vi "FIFO_96ch_Clear.vi"(3 "error in":errorcluster, 5 "FPGA VI Reference In":T1) -> (0 "error out":errorcluster, 2 "FPGA VI Reference Out":T1)   [LabVIEW 2011]
uses:
  FPGA_reference.ctl
  <vilib>/Utility/error.llb/Error Cluster From Error Code.vi
  <vilib>/rvi/errors/niLvFpgaAdjustHostInterfaceError.vi
  <vilib>/rvi/interface/nirviMethod/nirviMethod.xnode
  FPGA Bitfiles/FPGA96chmodular3_FPGATarget_fpga8ch-Main_90409DC7.lvbitx
  fpga_8ch-Main.vi
  <vilib>/FPGAPlugInAG/PXI-7813R/niLvFpga_ReadFifo_PXI-7813R.vi
  <vilib>/rvi/errors/niLvFpgaMergeErrorWithErrorCode.vi
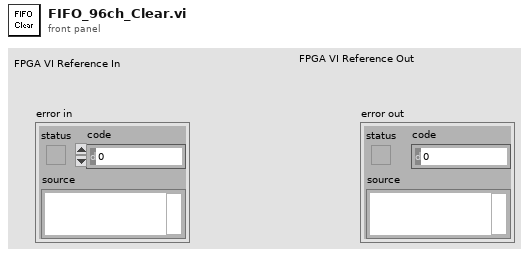
[diagram p1: front panel]
types:
  T1 = typedef "FPGA_reference.ctl" = refnum<k20>
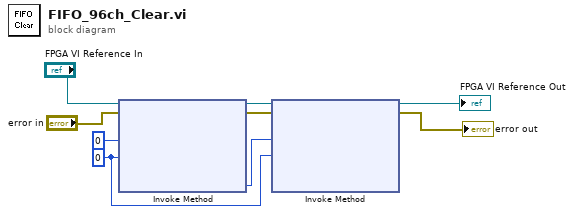
[diagram p0: block diagram]
diagram:
  w7 = 0 ("Timeout (ms)")
  n1 = xnode "Invoke Method"("FPGA VI Reference In"="FPGA VI Reference In", "error in"="error in", "Number of Elements"=u32 0, "Timeout (ms)"=w7) -> ("FPGA VI Reference Out"=w9:T1, "error out"=w4:errorcluster, "Elements Remaining"=w6:u32)  [unwired: 1 out]
  n2 = xnode "Invoke Method"("FPGA VI Reference In"=w9, "error in"=w4, "Number of Elements"=w6, "Timeout (ms)"=w7) -> ("FPGA VI Reference Out"=→"FPGA VI Reference Out":T1, "error out"=→"error out":errorcluster)  [unwired: 2 out]
